vi "7L24-pi_init_0.vi"(2 "Cc":dbl, 3 "T":dbl) -> (0 "Cc init":dbl, 1 "T init":dbl)   [LabVIEW 2010, in "lv_07.lvlib"]
uses:
  lv_07.lvlib
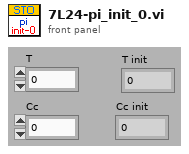
[diagram p1: front panel]
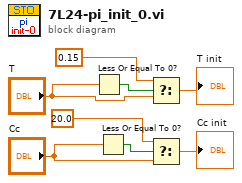
[diagram p0: block diagram]
diagram:
  n1 = Less Or Equal To 0?(x="T") -> (x <= 0?=w7:bool)
  n2 = Less Or Equal To 0?(x="Cc") -> (x <= 0?=w4:bool)
  n3 = Select(t=0.15 ("cas vrai"), s=w7, f="T") -> (s? t:f=→"T init":dbl)
  n4 = Select(t=20.0 ("cas vrai"), s=w4, f="Cc") -> (s? t:f=→"Cc init":dbl)
